vi "GetAngle.vi"(1 "Y-Value":dbl, 2 "X-Value":dbl) -> (0 "Angle":dbl)   [LabVIEW 2017]
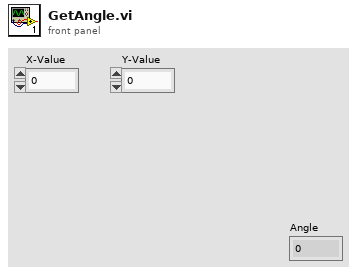
[diagram p1: front panel]
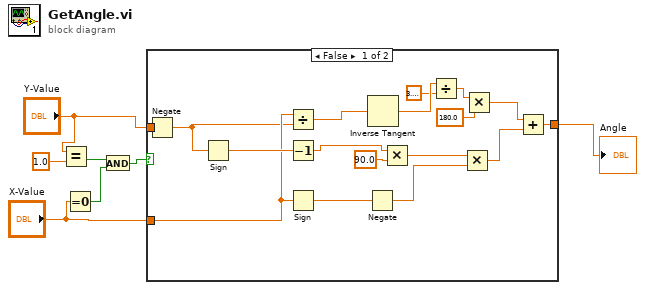
[diagram p0: block diagram]
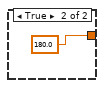
[diagram p2: hidden frame]
diagram:
  n1 = Equal?(x="Y-Value", y=1.0) -> (x = y?=w2:bool)
  n2 = Equal To 0?(x="X-Value") -> (x = 0?=w1:bool)
  n3 = And(x=w2, y=w1) -> (x .and. y?=w3:bool)
  n4 = case shown="False" w3 {
    tunnel: "Y-Value" -> [w22 _]
    tunnel: "X-Value" -> [w19 _]
    tunnel: [w17 180.0] -> w7
    frame False {
      n5 = Negate(x=w22) -> (-x=w8:dbl)
      n6 = Sign(1:w8) -> (0:w21:dbl)
      n7 = Divide(x=w19, y=w8) -> (x/y=w24:dbl)
      n8 = Decrement(x=w21) -> (x-1=w20:dbl)
      n9 = Sign(1:w19) -> (0:w18:dbl)
      n10 = Negate(x=w18) -> (-x=w16:dbl)
      n11 = Inverse Tangent(1:w24) -> (0:w11:dbl)
      n12 = Multiply(x=w20, y=90.0 ("x*y")) -> (x*y=w15:dbl)
      n13 = Divide(x=w11, y=3.141592653589793) -> (x/y=w12:dbl)
      n14 = Multiply(x=w15, y=w16) -> (x*y=w14:dbl)
      n15 = Multiply(x=w12, y=180.0) -> (x*y=w13:dbl)
      n16 = Add(x=w13, y=w14) -> (x+y=w17:dbl)
    }
    frame True {
    }
  }
  "Angle" <- w7
